vi "WSVCAP SHL Host LL I2C Build and Parse Write Message.vi"(0 "C1 Write Data In [DUT Ordered]":u8[][](array[numeric]) format="%.0x", 1 "Message In":string, 5 "C2 Write Data [DUT Ordered]":u8[][](array[numeric]) format="%.0x", 7 "C3Write Data [DUT Ordered]":u8[][](array[numeric]) format="%.0x", 9 "Socket Mask [U64] In":u64=1 format="%016x", 11 "error in":errorcluster, 12 "Sub Address In":u8=20 format="%.0x") -> (3 "Message Out":string, 4 "C1 Write Data Out [DUT Ordered]":u8[][](array[numeric]) format="%.0x", 6 "C2 Write Data Out [DUT Ordered]":u8[][](array[numeric]) format="%.0x", 8 "C3 Write Data Out [DUT Ordered]":u8[][](array[numeric]) format="%.0x", 10 "Socket Mask [U64] Out":u64=1 format="%08x", 14 "Sub Address Out":u8=20 format="%.0x", 15 "error out":errorcluster)   [LabVIEW 2012]
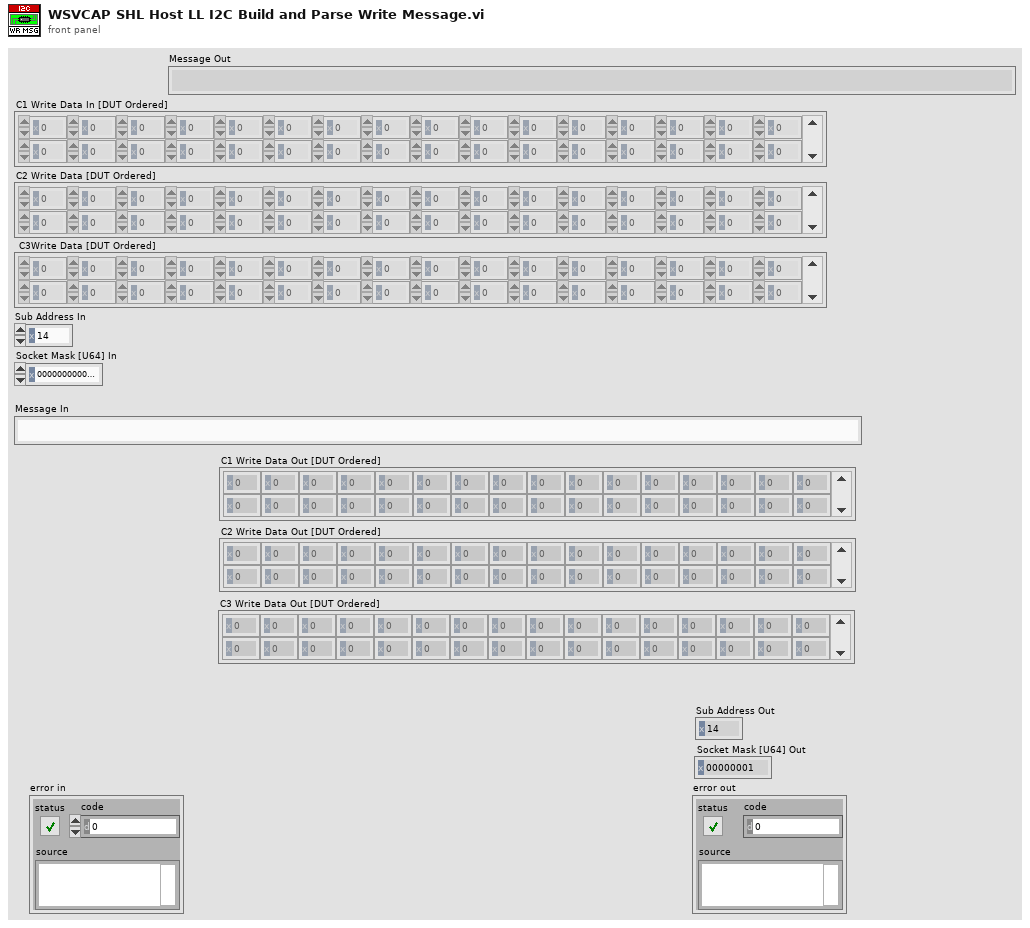
[diagram p1: front panel]
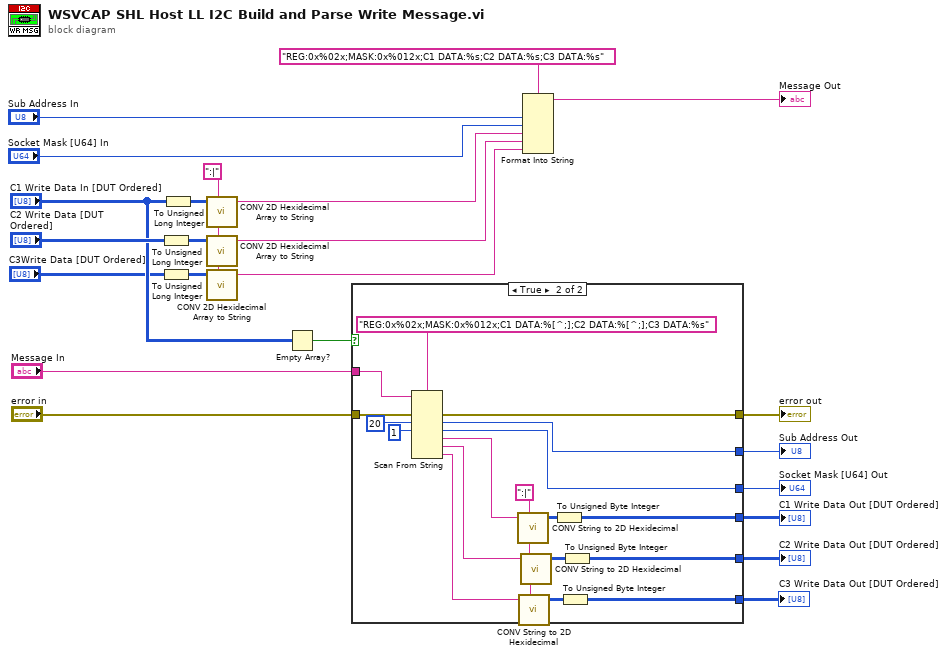
[diagram p0: block diagram]
diagram:
  w3 = ":|" ("Delimiters (,;)")
  n1 = To Unsigned Long Integer(number="C2 Write Data [DUT Ordered]") -> (unsigned 32bit integer=w5:u32[][])
  n2 = To Unsigned Long Integer(number="C3Write Data [DUT Ordered]") -> (unsigned 32bit integer=w6:u32[][])
  n3 = To Unsigned Long Integer(number="C1 Write Data In [DUT Ordered]") -> (unsigned 32bit integer=w23:u32[][])
  n4 = call "CONV 2D Hexidecimal Array to String.vi"("2-D Hexidecimal"=w23, "Delimiters (,;)"=w3) -> ("String"=w19:string)  [unwired: 7 in]
  n5 = call "CONV 2D Hexidecimal Array to String.vi"("2-D Hexidecimal"=w5, "Delimiters (,;)"=w3) -> ("String"=w18:string)  [unwired: 7 in]
  n6 = call "CONV 2D Hexidecimal Array to String.vi"("2-D Hexidecimal"=w6, "Delimiters (,;)"=w3) -> ("String"=w2:string)  [unwired: 7 in]
  n7 = Empty Array?(array="C1 Write Data In [DUT Ordered]") -> (empty?=w7:bool)
  n8 = case shown="True" w7 {
    tunnel: [_ w40] -> w16
    tunnel: [_ w39] -> w15
    tunnel: [_ w37] -> w14
    tunnel: [_ w36] -> w13
    tunnel: "error in" -> [w24 w33]
    tunnel: [w24 w32] -> w10
    tunnel: "Message In" -> [_ w31]
    tunnel: [_ w25] -> w1
    frame False {
    }
    frame True {
      w26 = ":|" ("Delimiters (,;)")
      n9 = Scan From String(format string="REG:0x%02x;MASK:0x%012x;C1 DATA:%[^;];C2 DATA:%[^;];C3 DATA:%s", input string=w31, error in=w33, default 1=u8 20 ("Sub Address Out"), default 2=u64 1 ("Socket Mask [U32] Out")) -> (error out=w32:errorcluster, output 1=w37:u8, output 2=w36:u64, output 3=w35:string, output 4=w34:string, output 5=w27:string)  [unwired: 4 in, 2 out]
      n10 = call "CONV String to 2D Hexidecimal.vi"("String"=w35, "Delimiters (,;)"=w26) -> ("2-D Hexidecimal"=w42:u32[][])  [unwired: 7 in]
      n11 = call "CONV String to 2D Hexidecimal.vi"("String"=w27, "Delimiters (,;)"=w26) -> ("2-D Hexidecimal"=w28:u32[][])  [unwired: 7 in]
      n12 = call "CONV String to 2D Hexidecimal.vi"("String"=w34, "Delimiters (,;)"=w26) -> ("2-D Hexidecimal"=w41:u32[][])  [unwired: 7 in]
      n13 = To Unsigned Byte Integer(number=w42) -> (unsigned 8bit integer=w40:u8[][])
      n14 = To Unsigned Byte Integer(number=w28) -> (unsigned 8bit integer=w25:u8[][])
      n15 = To Unsigned Byte Integer(number=w41) -> (unsigned 8bit integer=w39:u8[][])
    }
  }
  "C1 Write Data Out [DUT Ordered]" <- w16
  "C2 Write Data Out [DUT Ordered]" <- w15
  "Sub Address Out" <- w14
  "Socket Mask [U64] Out" <- w13
  "error out" <- w10
  "C3 Write Data Out [DUT Ordered]" <- w1
  n16 = Format Into String(format string="REG:0x%02x;MASK:0x%012x;C1 DATA:%s;C2 DATA:%s;C3 DATA:%s", "Sub Address In", "Socket Mask [U64] In", w19, w18, w2) -> (resulting string=→"Message Out":string)  [unwired: 2 in, 1 out]
